vi "REWORK_listbox_set_values_and_recolor.vi"(7 "column_names":string[](array[string]), 8 "error_in":errorcluster, 10 "REPORT_GEAR_station":T1=12 caption="Station:" items=["ALL"=0, "Station 10"=10, "Station 20"=20, "Station 30"=30, "Station 40"=40, "Station 50"=50, "Station 60"=60, "Station 70"=70, "Station 80"=80, "Station 90"=90, "Station 100"=100, "Station 110"=110, "Station 120"=120, "Station 160"=165], 11 "REPORT_all_info":T2) -> (0 "error_out":errorcluster)   [LabVIEW 2019]
uses:
  REWORK_all_info.ctl
  MAIN/REWORK_header_data_display.ctl
  REWORK_gear_statuses.ctl
  REWORK_references.ctl
  REWORK_gear_station.ctl
  <vilib>/Utility/miscctls.llb/LVRowAndColumnTypeDef.ctl
  <vilib>/Utility/miscctls.llb/LVRowAndColumnUnsignedTypeDef.ctl
  <userlib>/_OpenG.lib/array/array.llb/Filter 1D Array with Scalar (String)__ogtk.vi
panel:
  # "GEAR INFO SUMMARY"
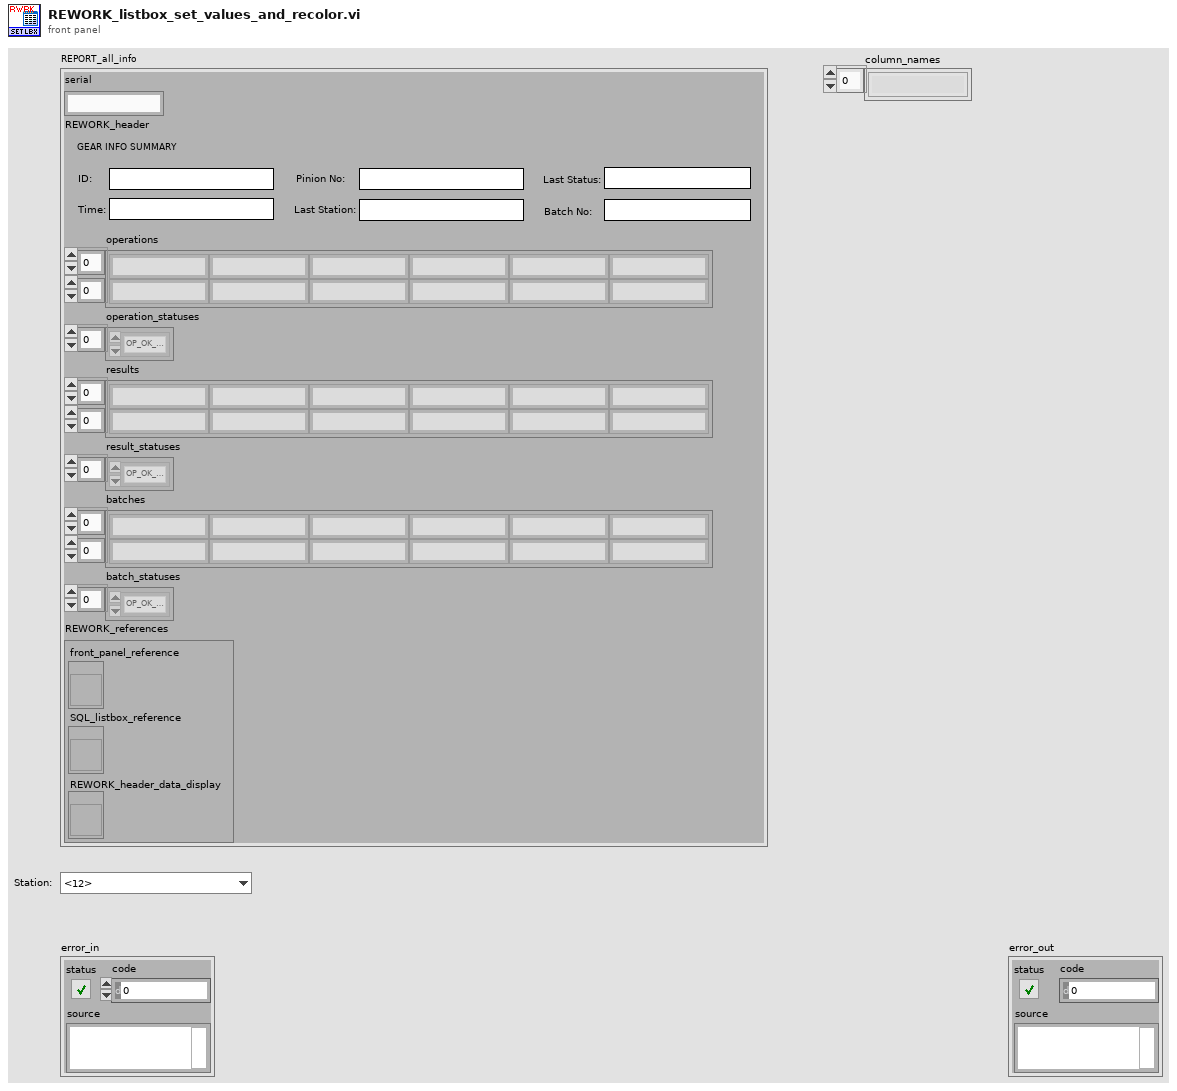
[diagram p1: front panel]
types:
  T1 = typedef "REWORK_gear_station.ctl" = u16
  T2 = typedef "REWORK_all_info.ctl" = cluster{"serial":string, "REWORK_header":T3, "operations":string[][], "operation_statuses":T4[], "results":string[][], "result_statuses":T4[], "batches":string[][], "batch_statuses":T4[], "REWORK_references":T5}
  T3 = typedef "REWORK_header_data_display.ctl" = cluster{"ID":string, "creation_time":string, "last_station":string, "last_status":string, "pinion_serial":string, "batch_code":string}
  T4 = typedef "REWORK_gear_statuses.ctl" = enum16{"OP_OK_hide", "OP_OK_show", "OP_NOK_hide", "OP_NOK_show", "OP_interrupted_hide", "OP_interrupted_show", "OP_in_operation_hide", "OP_in_operation_show", "OP_unexpected_hide", "OP_unexpected_show", "RE_REAL_OK", "RE_REAL_NOK", "RE_STRING", "RE_sub_header", "RE_no_data", "RE_unexpected", "BA_sub_header", "BA_data", "BA_no_data"}
  T5 = typedef "REWORK_references.ctl" = cluster{"front_panel_reference":refnum<vi>, "SQL_listbox_reference":refnum<vi>, "REWORK_header_data_display":refnum<vi>}
  T6 = typedef "LVRowAndColumnUnsignedTypeDef.ctl" = cluster{"Row":u32, "Column":u32}
  T7 = typedef "LVRowAndColumnTypeDef.ctl" = cluster{"Row":i32, "Column":i32}
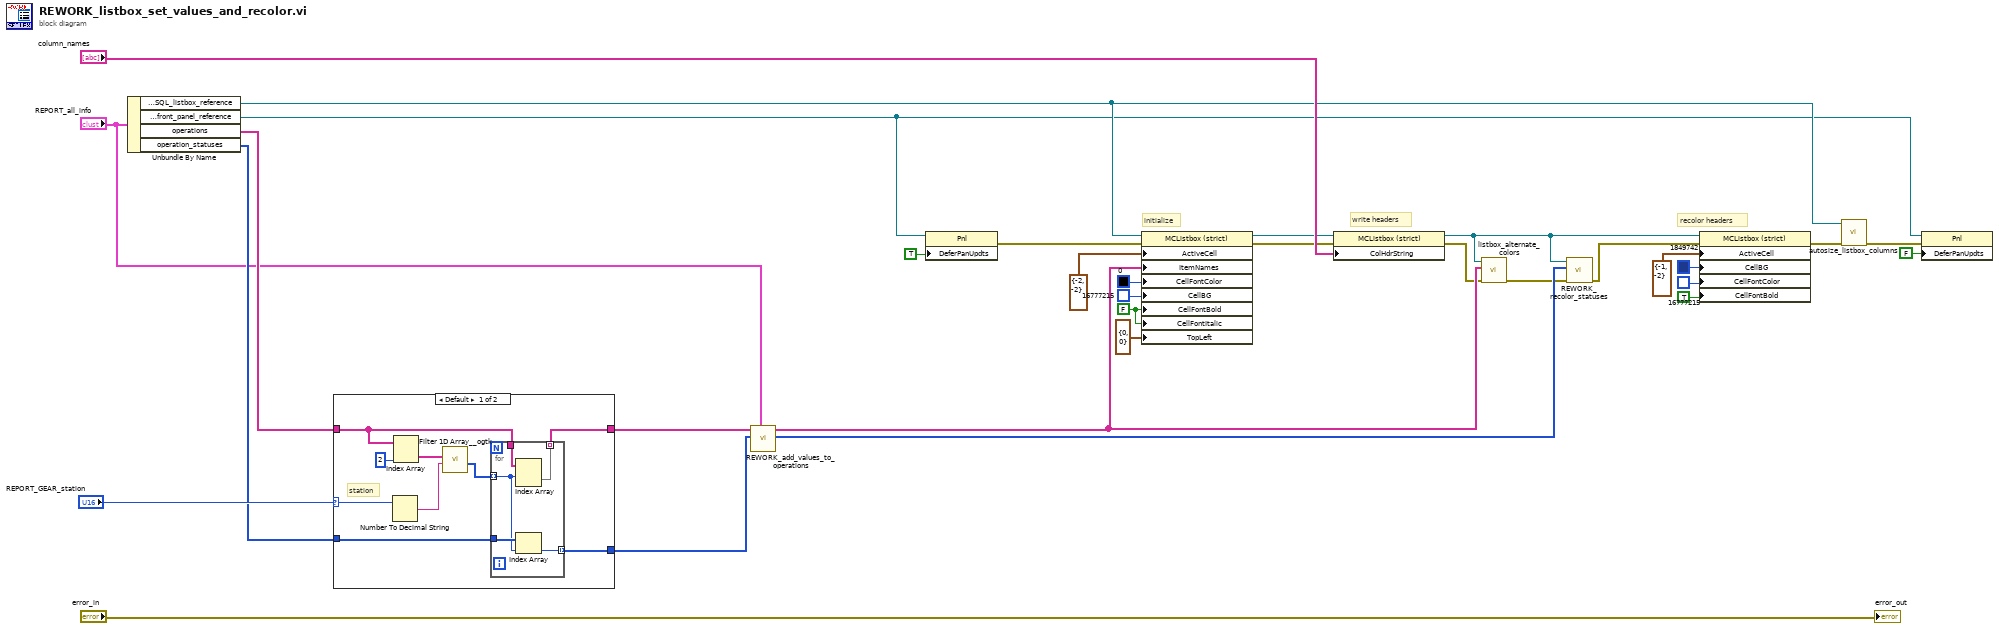
[diagram p0: block diagram]
diagram:
  w15 = FALSE ("Active Cell:Cell Font:Bold")
  # "recolor headers"
  # "initialize"
  # "write headers"
  n1 = Unbundle By Name("REPORT_all_info") -> ("REWORK_references.SQL_listbox_reference"=w23:refnum<vi>, "REWORK_references.front_panel_reference"=w22:refnum<vi>, "operations"=w20:string[][], "operation_statuses"=w19:T4[])
  n2 = case shown="Default" "REPORT_GEAR_station" {
    selector: "REPORT_GEAR_station" -> [w36 _]
    tunnel: w20 -> [w39 w48]
    tunnel: [w37 w48] -> w18
    tunnel: w19 -> [w34 w47]
    tunnel: [w33 w47] -> w17
    frame Default {
      # "station"
      n3 = Number To Decimal String(number=w36) -> (decimal integer string=w35:string)  [unwired: 1 in]
      n4 = Index Array(array=w39, index (col)=2 ("disabled index (col)")) -> (element=w40:string[])  [unwired: 1 in]
      n5 = call-poly <userlib>:"Filter 1D Array__ogtk.vi"("items to filter"=w35, "array"=w40) -> ("filtered item indices"=w38:i32[])  [unwired: 4 in, 1 out]
      n6 = for {
        tunnel: w39 -> [w46]
        tunnel: w38 -> [w43] mode=indexing
        tunnel: [w45] -> w37 mode=indexing
        tunnel: w34 -> [w44]
        tunnel: [w42] -> w33 mode=indexing
        n7 = Index Array(array=w46, index (row)=w43) -> (element=w45:string[])  [unwired: 1 in]
        n8 = Index Array(array=w44, index=w43) -> (element=w42:T4)
      }
    }
    frame 0 {
    }
  }
  n9 = call "REWORK_add_values_to_operations.vi"("REPORT_all_info"="REPORT_all_info", "operation_statuses"=w17, "operations"=w18) -> ("record_statuses"=w6:T4[], "ItemNames"=w12:string[][])  [unwired: 7 in]
  n10 = property on="Property Node" class="Pnl"(reference=w22, "DeferPanUpdts"=TRUE ("Defer Panel Updates")) -> (error out=w30:errorcluster)  [unwired: 1 in, 1 out]
  n11 = property on="Property Node" class="MCListbox (strict)"(reference=w23, error in=w30, "ActiveCell"=T7 {"Row"=-2, "Column"=-2} ("Active Cell:Active Cell"), "ItemNames"=w12, "CellFontColor"=u32 0, "CellBG"=u32 16777215, "CellFontBold"=w15, "CellFontItalic"=w15, "TopLeft"=T6 {"Row"=0, "Column"=0} ("Top Left Visible Cell")) -> (reference out=w26:refnum<vi>, error out=w24:errorcluster)
  n12 = property on="Property Node" class="MCListbox (strict)"(reference=w26, error in=w24, "ColHdrString"="column_names") -> (reference out=w7:refnum<vi>, error out=w4:errorcluster)
  n13 = call "listbox_alternate_colors.vi"("error_in"=w4, "item_names"=w12, "listbox_ref"=w7) -> ("error_out"=w5:errorcluster)  [unwired: 8 in]
  n14 = call "REWORK_recolor_statuses.vi"("error_in"=w5, "record_statuses"=w6, "listbox_ref"=w7) -> ("error_out"=w3:errorcluster)  [unwired: 8 in]
  n15 = property on="Property Node" class="MCListbox (strict)"(reference=w7, error in=w3, "ActiveCell"=T7 {"Row"=-1, "Column"=-2} ("Active Cell:Active Cell"), "CellBG"=u32 1849742, "CellFontColor"=u32 16777215, "CellFontBold"=TRUE ("Active Cell:Cell Font:Bold")) -> (error out=w29:errorcluster)  [unwired: 1 out]
  n16 = call "autosize_listbox_columns.vi"("error in (no error)"=w29, "Table Ref"=w23) -> ("error out"=w28:errorcluster)  [unwired: 4 in, 1 out]
  n17 = property on="Property Node" class="Pnl"(reference=w22, error in=w28, "DeferPanUpdts"=FALSE ("Defer Panel Updates")) -> ()  [unwired: 2 out]
  "error_out" <- "error_in"
